vi "Send WPL Command.vi"(8 "error in (no error)":errorcluster, 9 "Variant":variant, 10 "Command":T1, 11 "WPL Comm":refnum<class "WPL Comm.lvclass">) -> (0 "error out":errorcluster, 3 "WPL Comm Dup":refnum<class "WPL Comm.lvclass">)   [LabVIEW 2020, in "Internal Comm Classes.lvlib" / "WPL Comm.lvclass"]
uses:
  WPL Comm.lvclass
  WPL Command.ctl
  WPL Comm.lvclass/WPL Comm.ctl
  WPL Command Queue Cluster.ctl
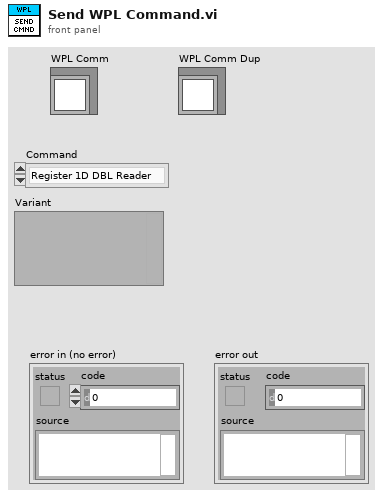
[diagram p1: front panel]
types:
  T1 = typedef "Internal Comm Classes.lvlib/WPL Comm.lvclass/WPL Command.ctl" = enum16{"Register 1D DBL Reader", "Unregister 1D DBL Reader", "Register 1D DBL Writer", "Register 2D DBL Writer", "Unregister 1D DBL Writer", "Unregister 2D DBL Writer", "DBL WFM Start", "WFM 1D DBL Data", "WFM 2D DBL Data", "Shut down", "Handle Error", "Register 1D CDB Reader", "Unregister 1D CDB Reader", "Register 1D CDB Writer", "Unregister 1D CDB Writer", "Register 2D CDB Writer", "Unregister 2D CDB Writer", "WFM 1D CDB Data", "WFM 2D CDB Data", "CDB WFM Start", "Error Shutdown", "Register Streams", "Unregister Streams", "Delete All Streams", "Get WFM DTs", "DBL WFM Multi Start", "CDB WFM Multi Start"}
  T2 = typedef "Internal Comm Classes.lvlib/WPL Comm.lvclass/WPL Command Queue Cluster.ctl" = cluster{"Command":T1, "Data":variant, "Idxs":i32[], "SampleOffset":u64}
  T3 = typedef "Internal Comm Classes.lvlib/WPL Comm.lvclass/Waveform error queue.ctl" = refnum<queue>
  T4 = typedef "Internal Comm Classes.lvlib/WPL Comm.lvclass/WPL Command Queue ref.ctl" = refnum<queue>
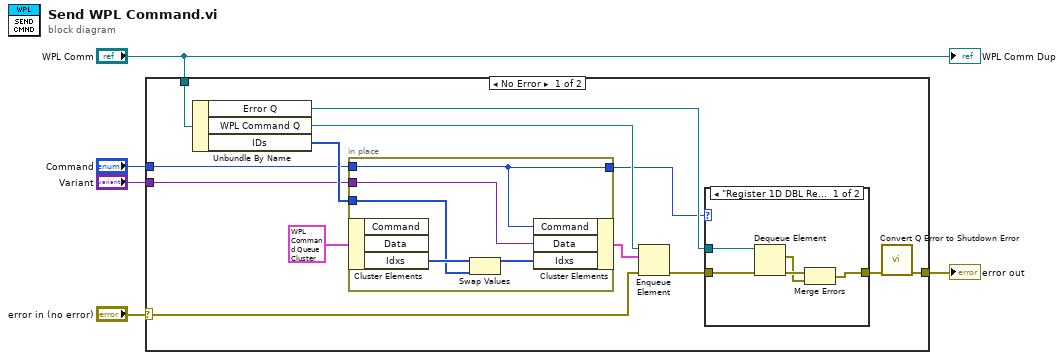
[diagram p0: block diagram]
diagram:
  n1 = case shown="No Error" "error in (no error)" {
    selector: "error in (no error)" -> [w6 w30]
    tunnel: "WPL Comm" -> [w17 _]
    tunnel: "Command" -> [w10 _]
    tunnel: "Variant" -> [w9 _]
    tunnel: [w7 w30] -> w2
    frame No Error {
      n2 = Unbundle By Name(w17) -> ("Error Q"=w16:T3, "WPL Command Q"=w15:T4, "IDs"=w14:i32[])
      n3 = in-place {
        in-place-border: w10 -> [w23]
        in-place-border: w9 -> [w22]
        in-place-border: w14 -> [w19]
        in-place-border: [w23] -> w12
        n4 = in-place-cluster #1(T2 {"Command"=enum."Register 1D DBL Reader", "Data"=variant, "Idxs"=[], "SampleOffset"=0} ("Queue Data")) -> ("Idxs"=w21:i32[])  [unwired: 2 out]
        n5 = Swap Values(12:w21, 14:w19) -> (1:w20:i32[])  [unwired: 1 in, 1 out]
        n6 = in-place-cluster #1("Command"=w23, "Data"=w22, "Idxs"=w20) -> (w11:T2)
      }
      n7 = Enqueue Element(queue=w15, element=w11, error in (no error)=w6) -> (error out=w18:errorcluster)  [unwired: 1 in, 2 out]
      n8 = case shown="\"Register 1D DBL Reader\"..\"Unregister 2D DBL Writer\", \"Register 1D CDB Reader\"..\"Unregister 2D CDB Writer\"" w12 {
        tunnel: w16 -> [w27 _]
        tunnel: w18 -> [w28 w29]
        tunnel: [w24 w29] -> w8
        frame "Register 1D DBL Reader".."Unregister 2D DBL Writer", "Register 1D CDB Reader".."Unregister 2D CDB Writer" {
          n9 = Dequeue Element(queue=w27, error in (no error)=w28) -> (element=w25:errorcluster, error out=w26:errorcluster)  [unwired: 1 in, 2 out]
          n10 = Merge Errors(w26, w25) -> (w24:errorcluster)
        }
        frame Default {
        }
      }
      n11 = call "Convert Q Error to Shutdown Error.vi"("error in (no error)"=w8) -> ("error out"=w7:errorcluster)  [unwired: 10 in]
    }
    frame Error {
    }
  }
  "error out" <- w2
  "WPL Comm Dup" <- "WPL Comm"
